vi "WaitPassSkill.vi"(6 "Best Y Inverso":dbl[](array[numeric]), 8 "error in (no error)":errorcluster, 9 "Game":refnum<class "Game.lvclass">, 10 "Robot":refnum<class "Robot.lvclass">, 11 "WaitPassSkill in":refnum<class "WaitPassSkill.lvclass">) -> (0 "error out":errorcluster, 2 "Robot out":refnum<class "Robot.lvclass">, 3 "WaitPassSkill out":refnum<class "WaitPassSkill.lvclass">)   [LabVIEW 2023, in "WaitPassSkill.lvclass"]
uses:
  WaitPassSkill.lvclass
  Robot_class/Robot.lvclass
  C:/Users/roboi/Downloads/VSS_AI-Larc2023 - Copia (2)/Object_class/Object.lvclass
  Game_class/Game.lvclass
  Utilities_class/Utilities.lvclass
  Object_class/Object.lvclass/Object.ctl
  Game_class/Game.lvclass/Game.ctl
  Ball_class/Ball.lvclass/Ball.ctl
  Team_class/Team.lvclass/Team.ctl
  Robot_class/roles.ctl
  Robot_class/Robot.lvclass/Robot.ctl
  Robot_class/Read role.vi
  Object_class/Read x.vi
  Object_class/Read y.vi
  <vilib>/Analysis/_algsub.llb/Real Vector Norm.vi
  Robot_class/Write dest_x.vi
  Robot_class/Write dest_y.vi
  Robot_class/Write dest_orientation.vi
  Robot_class/Write dest_vel.vi
  Game_class/Read BallRef.vi
  Game_class/Read OffensiveTeam.vi
  Team_class/Read RobotRef.vi
  Ball_class/Read v_x.vi
  Ball_class/Read v_y.vi
  Robot_class/Write dest_x_kick.vi
  Robot_class/Write dest_y_kick.vi
  Ally_class/Ally.lvclass
  C:/Users/roboi/Downloads/VSS_AI-Larc2023 - Copia (2)/Team_class/Team.lvclass
  Ball_class/Ball.lvclass
  <vilib>/Analysis/NI_AALPro.lvlib
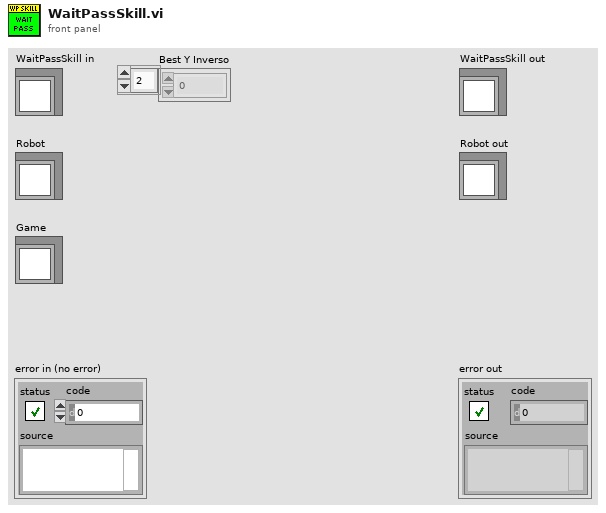
[diagram p1: front panel]
types:
  T1 = typedef "roles.ctl" = enum16{"BallChallengerAttackerVSS", "NormalAttackerVSS", "AttackerAimGoalVSS", "DefenderAreaVSS", "KeeperVSS", "Tabler", "TableFinalizer", "PrepareRollToPassRoller", "PrepareRollToPassReceiver", "SimplePassRoll", "SimplePassRollReceiver", "PenaltyDefense", "PreparePassReceiver 2", "PreparePassReceiver 1", "PassObserver", "Timeout", "Goto", "ZigZag", "None", "BallOutOfField", "DefenderArea", "Duelist", "AttackerStop", "FollowAttacker", "KeeperRole", "KickPenalty", "AttackerAimGoal", "AttackerBlock", "Marker", "Halt", "Shoot", "PassKicker", "PassReceiver", "TestRole", "PenaltyAttacker"}
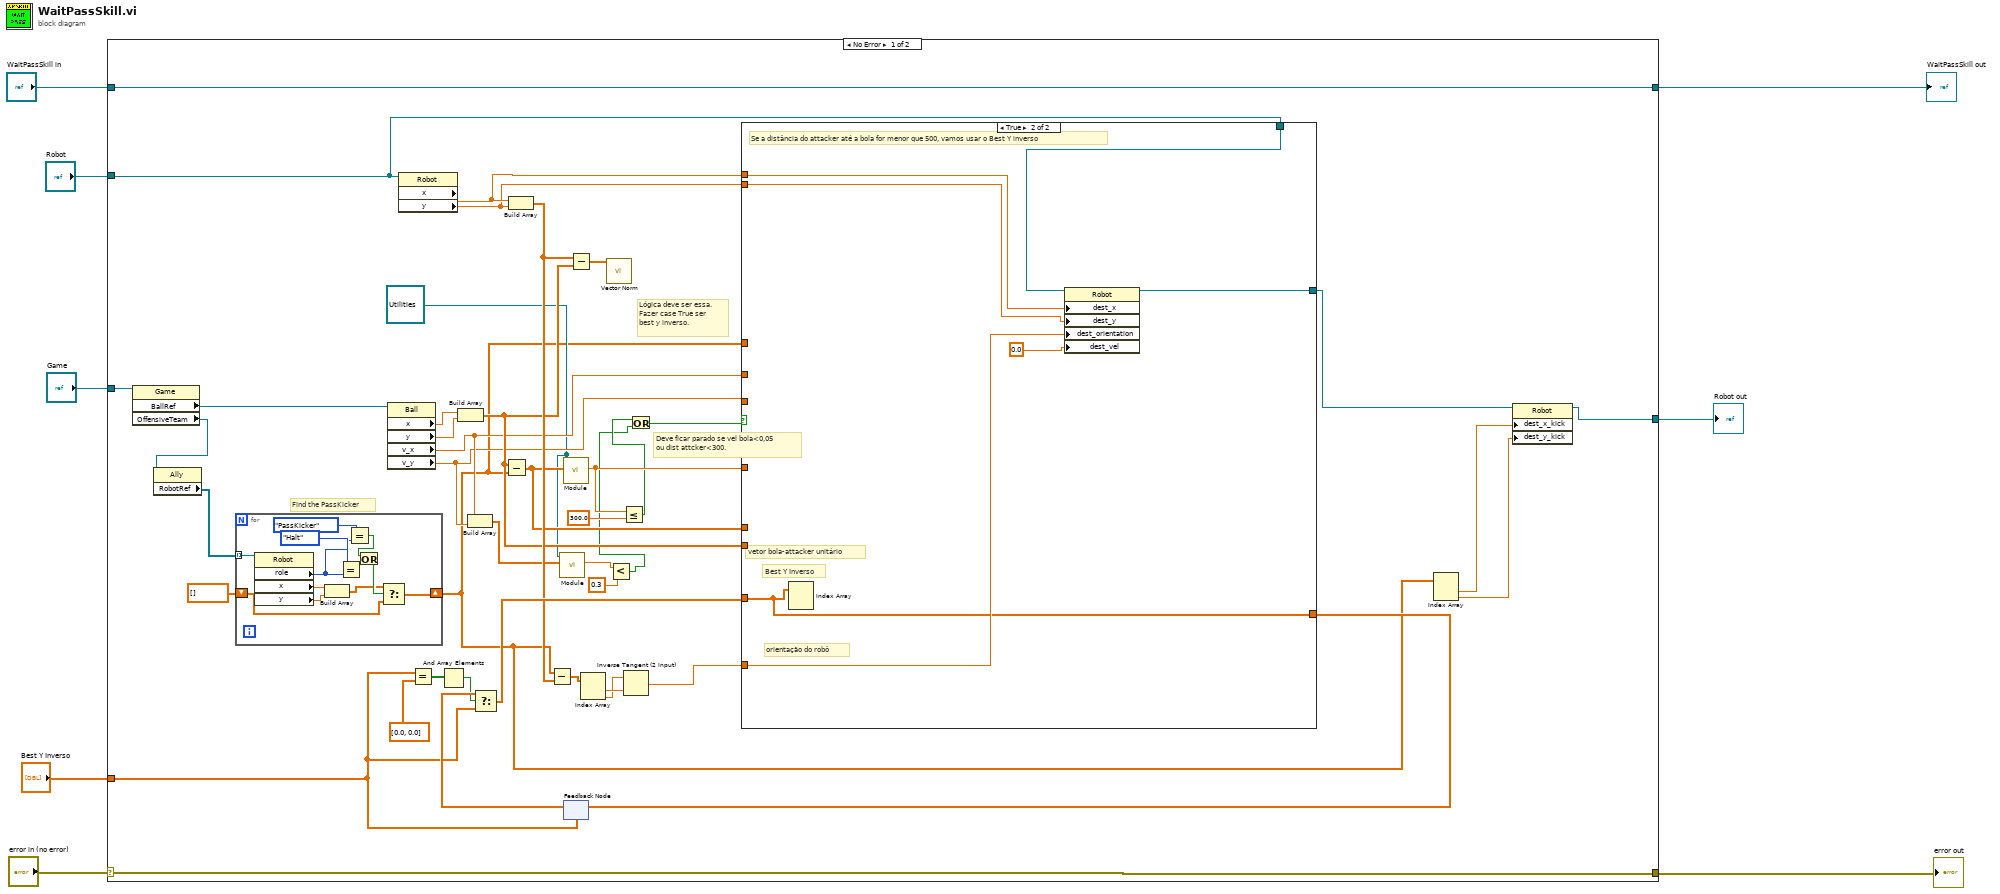
[diagram p0: block diagram]
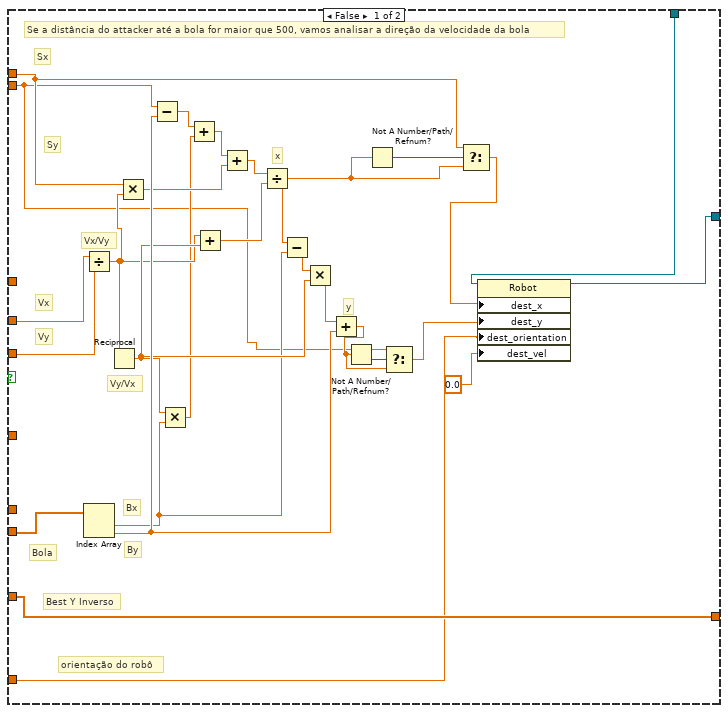
[diagram p2: hidden frame]
diagram:
  n1 = case shown="No Error" "error in (no error)" {
    selector: "error in (no error)" -> [w50 w101]
    tunnel: [w50 w101] -> w7
    tunnel: [w51 w100] -> w5
    tunnel: "WaitPassSkill in" -> [w51 w100]
    tunnel: "Robot" -> [w14 w99]
    tunnel: "Game" -> [w28 _]
    tunnel: "Best Y Inverso" -> [w27 _]
    tunnel: [w26 w99] -> w1
    frame No Error {
      w17 = refnum<class "Utilities.lvclass"> refnum ("Utilities in")
      # "Lógica deve ser essa.\nFazer case True ser\nbest y inverso."
      # "Deve ficar parado se vel bola<0,05\nou dist attcker<300."
      # "Find the PassKicker"
      n2 = property class="Game"(reference=w28) -> ("BallRef"=w34:refnum<class "Ball.lvclass">, "OffensiveTeam"=w23:refnum<class "Ally.lvclass">)  [unwired: 1 in, 2 out]
      n3 = property class="Ally"(reference=w23) -> ("RobotRef"=w22:refnum<class "Robot.lvclass">[])  [unwired: 1 in, 2 out]
      n4 = for {
        tunnel: w22 -> [w63] mode=indexing
        shift-right: [w52] -> w15
        shift-left: dbl[] [] -> [w53]
        n5 = property class="Robot"(reference=w63) -> ("role"=w59:T1, "x"=w56:dbl, "y"=w55:dbl)  [unwired: 1 in, 2 out]
        n6 = Build Array(w56, w55) -> (w54:dbl[])
        n7 = Equal?(x=roles."Halt", y=w59) -> (x = y?=w61:bool)
        n8 = Equal?(x=roles."PassKicker", y=w59) -> (x = y?=w60:bool)
        n9 = Or(x=w60, y=w61) -> (x .or. y?=w57:bool)
        n10 = Select(t=w54, s=w57, f=w53) -> (s? t:f=w52:dbl[])
      }
      n11 = property class="Ball"(reference=w34) -> ("x"=w33:dbl, "y"=w32:dbl, "v_x"=w20:dbl, "v_y"=w19:dbl)  [unwired: 1 in, 2 out]
      n12 = property class="Robot"(reference=w14) -> ("x"=w36:dbl, "y"=w35:dbl)  [unwired: 1 in, 2 out]
      n13 = Equal?(x=w27, y=dbl[] [0.0, 0.0] ("FinalPosition")) -> (x = y?=w41:bool[])
      n14 = And Array Elements(Boolean array=w41) -> (logical AND=w40:bool)
      n15 = Build Array(w33, w32) -> (w38:dbl[])
      n16 = Build Array(w20, w19) -> (w18:dbl[])
      n17 = Subtract(x=w38, y=w15) -> (x-y=w25:dbl[])
      n18 = Build Array(w36, w35) -> (w39:dbl[])
      n19 = Subtract(x=w15, y=w39) -> (x-y=w47:dbl[])
      n20 = call "Module.vi"("2D vector"=w18, "Utilities in"=w17) -> ("Modulo"=w11:dbl)  [unwired: 7 in, 2 out]
      n21 = call "Module.vi"("2D vector"=w25, "Utilities in"=w17) -> ("Modulo"=w24:dbl)  [unwired: 7 in, 2 out]
      n22 = feedback #1(w27) -> (w43:dbl[])
      n23 = Select(t=w43, s=w40, f=w27) -> (s? t:f=w42:dbl[])
      n24 = Subtract(x=w39, y=w38) -> (x-y=w37:dbl[])
      n25 = Index Array(array=w47) -> (element #1=w49:dbl, element #2=w48:dbl)  [unwired: 2 in]
      n26 = call-poly <vilib>:"Vector Norm.vi"("Input Vector"=w37) -> ()  [unwired: 9 in, 2 out]
      n27 = Less?(x=w11, y=0.3) -> (x < y?=w10:bool)
      n28 = Less Or Equal?(x=w24, y=300.0) -> (x <= y?=w13:bool)
      n29 = Inverse Tangent (2 Input)(1:w49, 2:w48) -> (0:w46:dbl)
      n30 = Or(x=w13, y=w10) -> (x .or. y?=w9:bool)
      n31 = case shown="True" w9 {
        tunnel: w36 -> [w67 w93]
        tunnel: w35 -> [w64 w92]
        tunnel: w25 -> [_ _]
        tunnel: w24 -> [_ _]
        tunnel: w15 -> [_ _]
        tunnel: w46 -> [w74 w98]
        tunnel: w20 -> [w79 _]
        tunnel: w19 -> [w78 _]
        tunnel: w38 -> [w77 _]
        tunnel: w42 -> [w76 w95]
        tunnel: [w76 w95] -> w45
        tunnel: w14 -> [w75 w97]
        tunnel: [w72 w96] -> w31
        frame False {
          # "y"
          # "x"
          # "Vy/Vx"
          # "Vx/Vy"
          # "By"
          # "Bx"
          # "Best Y Inverso"
          # "Bola"
          # "Vy"
          # "Vx"
          # "orientação do robô"
          # "Sy"
          # "Sx"
          # "Se a distância do attacker até a bola for maior que 500, vamos analisar a direção da velocidade da bola"
          n32 = Divide(x=w79, y=w78) -> (x/y=w84:dbl)
          n33 = Index Array(array=w77) -> (element #1=w87:dbl, element #2=w91:dbl)  [unwired: 2 in]
          n34 = Reciprocal(x=w84) -> (1/x=w89:dbl)
          n35 = Multiply(x=w67, y=w84) -> (x*y=w83:dbl)
          n36 = Subtract(x=w64, y=w91) -> (x-y=w80:dbl)
          n37 = Multiply(x=w89, y=w87) -> (x*y=w81:dbl)
          n38 = Add(x=w80, y=w81) -> (x+y=w82:dbl)
          n39 = Add(x=w84, y=w89) -> (x+y=w86:dbl)
          n40 = Add(x=w82, y=w83) -> (x+y=w85:dbl)
          n41 = Divide(x=w85, y=w86) -> (x/y=w70:dbl)
          n42 = Subtract(x=w70, y=w87) -> (x-y=w88:dbl)
          n43 = Multiply(x=w88, y=w89) -> (x*y=w90:dbl)
          n44 = Add(x=w90, y=w91) -> (x+y=w66:dbl)
          n45 = Not A Number/Path/Refnum?(number/path/refnum=w66) -> (NaN/Path/Refnum?=w68:bool)
          n46 = Not A Number/Path/Refnum?(number/path/refnum=w70) -> (NaN/Path/Refnum?=w71:bool)
          n47 = Select(t=w64, s=w68, f=w66) -> (s? t:f=w65:dbl)
          n48 = Select(t=w67, s=w71, f=w70) -> (s? t:f=w69:dbl)
          n49 = property class="Robot"(reference=w75, "dest_x"=w69, "dest_y"=w65, "dest_orientation"=w74, "dest_vel"=0.0) -> (reference out=w72:refnum<class "Robot.lvclass">)  [unwired: 1 in, 1 out]
        }
        frame True {
          # "Best Y Inverso"
          # "Se a distância do attacker até a bola for menor que 500, vamos usar o Best Y inverso"
          # "orientação do robô"
          # "vetor bola-attacker unitário"
          n50 = Index Array(array=w95) -> ()  [unwired: 2 in, 2 out]
          n51 = property class="Robot"(reference=w97, "dest_x"=w93, "dest_y"=w92, "dest_orientation"=w98, "dest_vel"=0.0 ("dest_orientation")) -> (reference out=w96:refnum<class "Robot.lvclass">)  [unwired: 1 in, 1 out]
        }
      }
      n52 = feedback-in #1(w45) -> ()
      n53 = Index Array(array=w15) -> (element #1=w30:dbl, element #2=w29:dbl)  [unwired: 2 in]
      n54 = property class="Robot"(reference=w31, "dest_x_kick"=w30, "dest_y_kick"=w29) -> (reference out=w26:refnum<class "Robot.lvclass">)  [unwired: 1 in, 1 out]
    }
    frame Error {
    }
  }
  "error out" <- w7
  "WaitPassSkill out" <- w5
  "Robot out" <- w1
